vi "Matlab Script.vi"(6 "Marker_Size":string, 7 "nom source":string, 8 "error in":errorcluster, 9 "path to matlab":path, 10 "Color of points":string, 11 "style of points":string) -> (0 "error out":errorcluster, 3 "path":path)   [LabVIEW 2023]
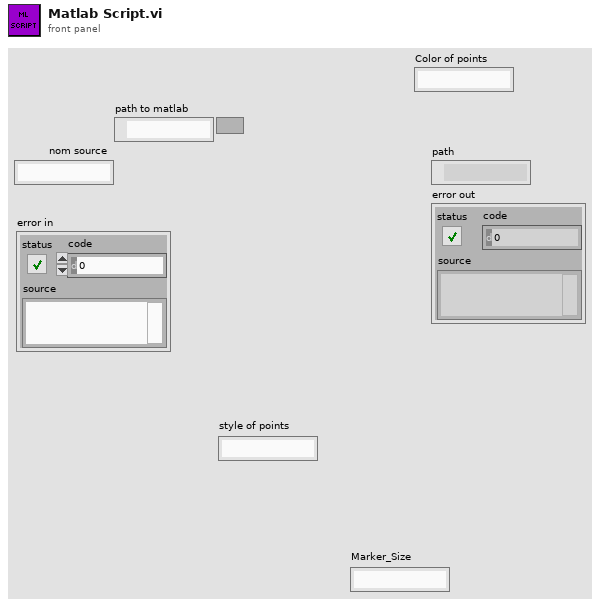
[diagram p1: front panel]
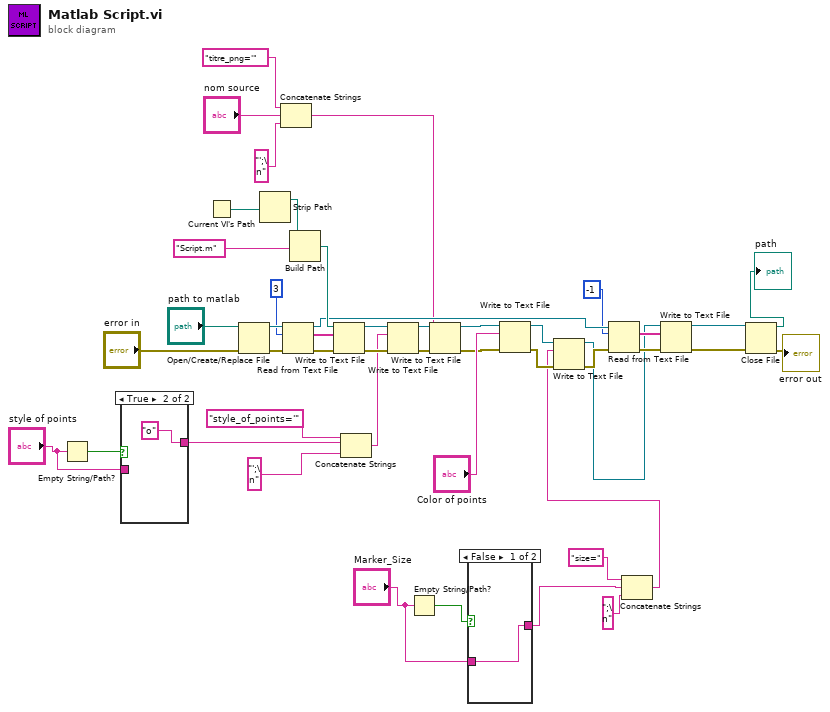
[diagram p0: block diagram]
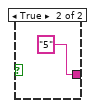
[diagram p2: hidden frame]
diagram:
  n1 = Empty String/Path?(string/path="style of points") -> (empty?=w21:bool)
  n2 = case shown="True" w21 {
    tunnel: [w47 "o"] -> w20
    tunnel: "style of points" -> [w47 _]
    frame False {
    }
    frame True {
    }
  }
  n3 = Current VI's Path() -> (path=w37:path)
  n4 = Open/Create/Replace File(file path (use dialog)="path to matlab", error in="error in") -> (refnum out=w45:refnum<file>, error out=w44:errorcluster)  [unwired: 4 in, 1 out]
  n5 = Strip Path(path=w37) -> (stripped path=w36:path)  [unwired: 1 out]
  n6 = Concatenate Strings("titre_png='" ("string"), "nom source", "';\n" ("string")) -> (w11:string)
  n7 = Read from Text File(file (use dialog)=w45, count=3, error in=w44) -> (refnum out=w27:refnum<file>, text=w41:string[], error out=w40:errorcluster)  [unwired: 1 in, 1 out]
  n8 = Build Path(base path=w36, name or relative path="Script.m") -> (appended path=w34:path)
  n9 = Write to Text File(file (use dialog)=w34, text=w41, error in=w40) -> (refnum out=w32:refnum<file>, error out=w33:errorcluster)  [unwired: 1 in, 1 out]
  n10 = Concatenate Strings("style_of_points='" ("string"), w20, "';\n" ("string")) -> (w29:string)
  n11 = Write to Text File(file (use dialog)=w32, text=w29, error in=w33) -> (refnum out=w17:refnum<file>, error out=w16:errorcluster)  [unwired: 1 in, 1 out]
  n12 = Empty String/Path?(string/path="Marker_Size") -> (empty?=w3:bool)
  n13 = Write to Text File(file (use dialog)=w17, text=w11, error in=w16) -> (refnum out=w18:refnum<file>, error out=w15:errorcluster)  [unwired: 1 in, 1 out]
  n14 = case shown="False" w3 {
    tunnel: [w49 "5"] -> w2
    tunnel: "Marker_Size" -> [w49 _]
    frame False {
    }
    frame True {
    }
  }
  n15 = Write to Text File(file (use dialog)=w18, text="Color of points", error in=w15) -> (refnum out=w8:refnum<file>, error out=w10:errorcluster)  [unwired: 1 in, 1 out]
  n16 = Concatenate Strings("size=" ("string"), w2, ";\n" ("string")) -> (w4:string)
  n17 = Write to Text File(file (use dialog)=w8, text=w4, error in=w10) -> (refnum out=w7:refnum<file>, error out=w9:errorcluster)  [unwired: 1 in, 1 out]
  n18 = Read from Text File(file (use dialog)=w27, count=-1, error in=w9) -> (text=w24:string[], error out=w25:errorcluster)  [unwired: 1 in, 2 out]
  n19 = Write to Text File(file (use dialog)=w7, text=w24, error in=w25) -> (refnum out=w22:refnum<file>, error out=w23:errorcluster)  [unwired: 1 in, 1 out]
  n20 = Close File(refnum=w22, error in=w23) -> (path=→"path":path, error out=→"error out":errorcluster)
